vi "9.2. загрузка параметров натекания.vi"() -> (2 "path param":path, 3 "param_out":dbl[](array[numeric]))   [LabVIEW 2016, in "Library.lvlib"]
uses:
  <vilib>/Utility/file.llb/Read From Spreadsheet File (DBL).vi
  <vilib>/Utility/file.llb/Write To Spreadsheet File (string).vi
  Granule-2000AT/PC/Library.lvlib
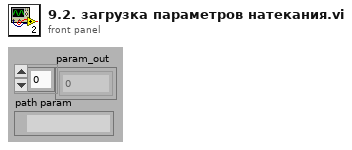
[diagram p1: front panel]
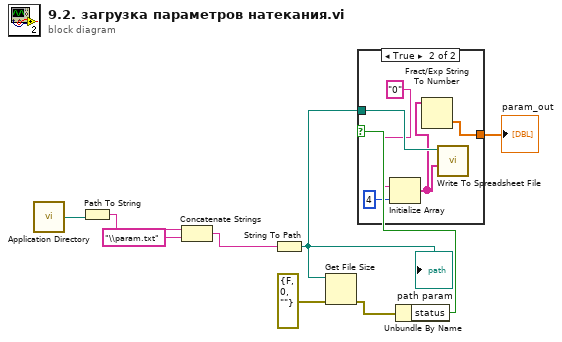
[diagram p0: block diagram]
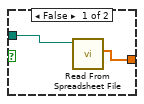
[diagram p2: hidden frame]
diagram:
  n1 = call <vilib>:"Application Directory.vi"() -> ("Application Directory"=w9:path)
  n2 = Path To String(path=w9) -> (string=w8:string)
  n3 = Concatenate Strings(w8, "\\param.txt" ("string")) -> (w6:string)
  n4 = String To Path(string=w6) -> (path=w2:path)
  "path param" <- w2
  n5 = Get File Size(file=w2, error in=errorcluster {"status"=FALSE, "code"=0, "source"=""}) -> (0:w4:errorcluster)  [unwired: 2 out]
  n6 = Unbundle By Name(w4) -> ("status"=w3:bool)
  n7 = case shown="True" w3 {
    tunnel: w2 -> [w10 w16]
    tunnel: [w11 w12] -> w1
    frame False {
      n8 = call-poly <vilib>:"Read From Spreadsheet File.vi"("file path (dialog if empty)"=w10) -> ("first row"=w11:dbl[])  [unwired: 6 in, 4 out]
    }
    frame True {
      n9 = Initialize Array("0", 4 ("dimension size")) -> (w13:string[])
      n10 = Fract/Exp String To Number(string=w13) -> (number=w12:dbl[])  [unwired: 3 in, 1 out]
      n11 = call-poly <vilib>:"Write To Spreadsheet File.vi"("1D data"=w13, "file path (dialog if empty)"=w16) -> ()  [unwired: 6 in, 1 out]
    }
  }
  "param_out" <- w1
